vi "Melissa.vi"(9 "REPL":string, 10 "Send":string) -> ()   [LabVIEW 2020]
panel:
  in  "Serial Name":string
  out "Cover":bool
  in  "Script":string
  in  "Buffer":string
  in  "Disconnect":bool
  in  "Help":bool
  in  "Connect":bool
  in  "Stop Button":bool
  out "Running Script":bool
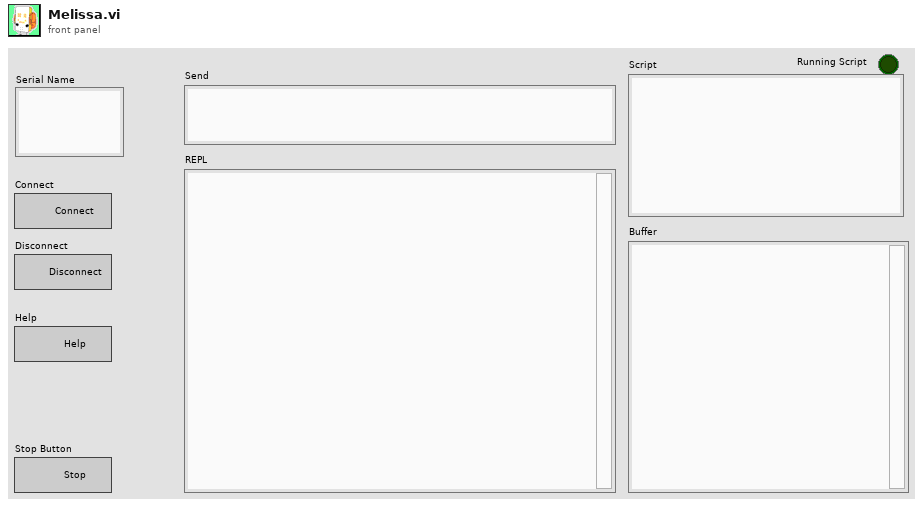
[diagram p1: front panel]
types:
  T1 = enum32{"Invalid", "Standard", "Closed", "Hidden", "Minimized", "Maximized"}
  T2 = typedef "eventvkey.ctl" = enum16{"ASCII", "Enter", "Return", "Shift", "Ctrl", "Alt", "Cmd", "Opt", "Caps", "NumLock", "Clear", "Break", "Up", "Down", "Left", "Right", "Insert", "Delete", "Home", "End", "PageUp", "PageDown", "Escape", "Help", "Pause", "ScrollLock", "F1", "F2", "F3", "F4", "F5", "F6", "F7", "F8", "F9", "F10", "F11", "F12", "F13", "F14", "F15", "F16", "F17", "F18", "F19", "F20", "F21", "F22", "F23", "F24", "Play", "VolumeUp", "VolumeDown", "Mute", "Two Byte Char"}
  T3 = cluster{"Shift":bool, "Ctrl":bool, "Alt":bool, "Cmd":bool, "Opt":bool}
  T4 = cluster{"Char":i16, "VKey":T2, "PlatMods":cluster{"Shift":bool, "Ctrl":bool, "Alt":bool, "Cmd":bool, "Opt":bool}}
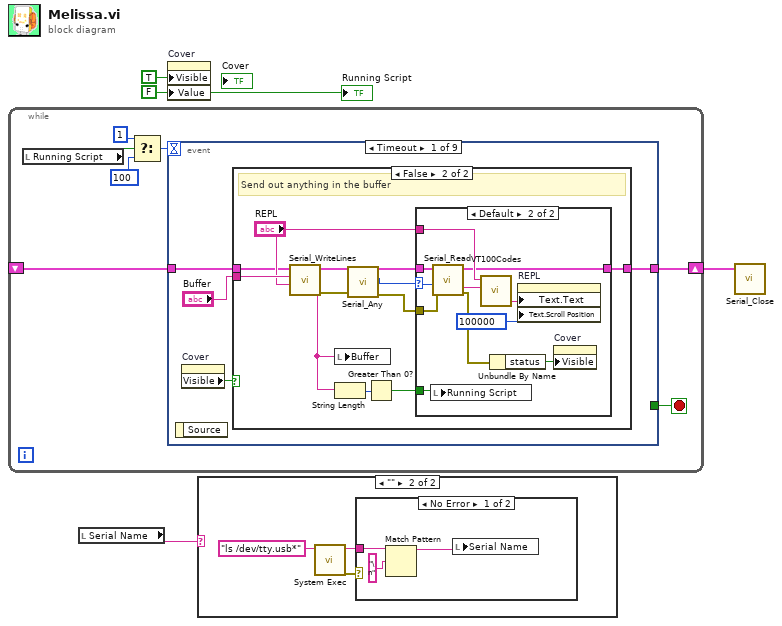
[diagram p0: block diagram]
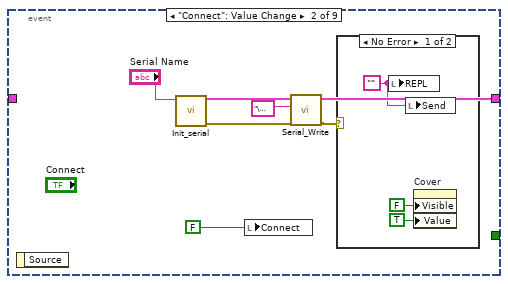
[diagram p6: hidden frame]
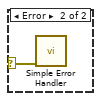
[diagram p7: hidden frame]
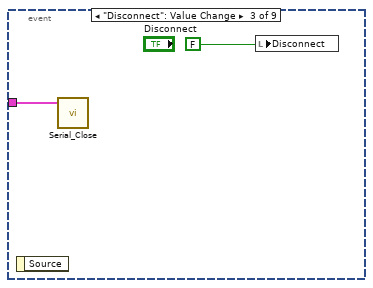
[diagram p8: hidden frame]
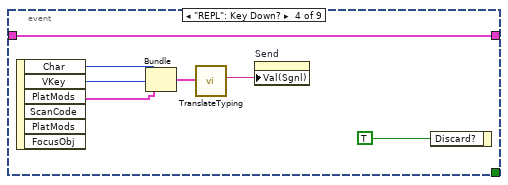
[diagram p9: hidden frame]
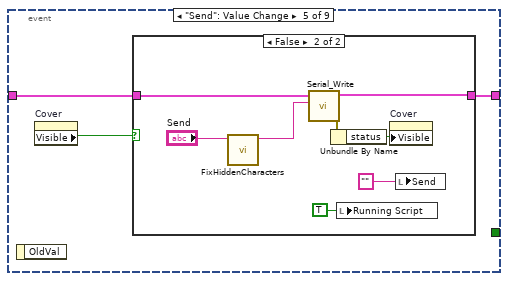
[diagram p10: hidden frame]
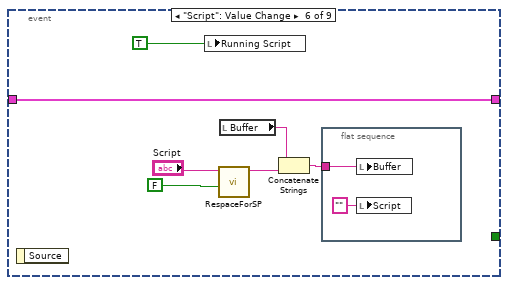
[diagram p12: hidden frame]
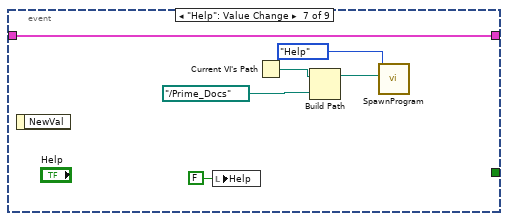
[diagram p13: hidden frame]
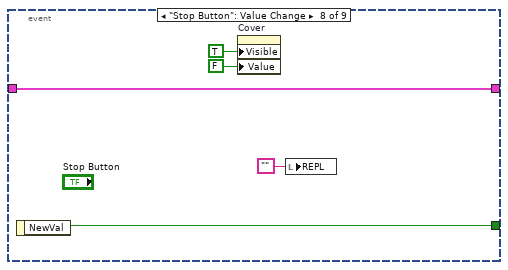
[diagram p14: hidden frame]
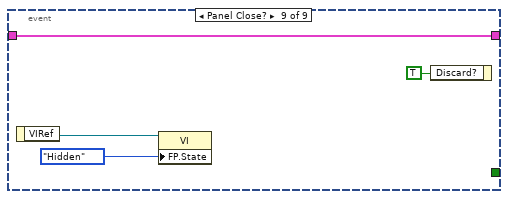
[diagram p15: hidden frame]
diagram:
  w3 = FALSE ("Cover")
  n1 = while {
    shift-right: [w10] -> w2
    shift-left: _ -> [w9]
    stop <- w11 stop-if-true
    n2 = local read "Running Script"() -> (w5:bool)
    n3 = Select(t=1, s=w5, f=100) -> (s? t:f=w6:i32)
    n4 = event shown="[0] Timeout" {
      selector: _ -> [_ _ _ _ _ _ _ _ _]
      dyn-events: _ -> [_ _ _ _ _ _ _ _ _]
      timeout: w6 -> [_ _ _ _ _ _ _ _ _]
      tunnel: [_ _ _ _ _ _ _ w90 _] -> w11
      tunnel: [w15 w41 _ w60 w62 w77 w87 w91 w96] -> w10
      tunnel: w9 -> [w14 _ w52 w60 w63 w77 w87 w91 w96]
      event Timeout {
        n5 = event-data() -> ()  [unwired: 1 in, 1 out]
        n6 = property on="Cover" class="Bool (strict)"() -> ("Visible"=w13:bool)  [unwired: 2 in, 2 out]
        n7 = case shown="False" w13 {
          tunnel: [w16 w18] -> w15
          tunnel: w14 -> [w16 w17]
          tunnel: "Buffer" -> [_ w28]
          frame True {
          }
          frame False {
            # "Send out anything in the buffer"
            n8 = call "Serial_WriteLines.vi"("REPL"="REPL", "Send"=w28, "Python in"=w17) -> ("error out"=w21:errorcluster, "Rest"=w26:string, "Python out"=w23:cluster{"Python":refnum<k35>, "py file":path})  [unwired: 6 in]
            n9 = local write "Buffer"(w26) -> ()
            n10 = String Length(string=w26) -> (length=w27:i32)
            n11 = call "Serial_Any.vi"("error in (no error)"=w21, "Python in"=w23) -> ("error out"=w20:errorcluster, "Size"=w19:i32, "Python out"=w22:cluster{"Python":refnum<k35>, "py file":path})  [unwired: 6 in, 1 out]
            n12 = Greater Than 0?(x=w27) -> (x > 0?=w25:bool)
            n13 = case shown="Default" w19 {
              selector: w19 -> [_ w30]
              tunnel: [w29 w34] -> w18
              tunnel: w22 -> [w29 w35]
              tunnel: w20 -> [_ w33]
              tunnel: w25 -> [_ w37]
              tunnel: "REPL" -> [_ w36]
              frame 0 {
              }
              frame Default {
                n14 = local write "Running Script"(w37) -> ()
                n15 = call "Serial_Read.vi"("error in (no error)"=w33, "Bytes"=w30, "Python in"=w35) -> ("error out"=w32:errorcluster, "text read"=w31:string, "Python out"=w34:cluster{"Python":refnum<k35>, "py file":path})  [unwired: 6 in]
                n16 = call "VT100Codes.vi"("read buffer"=w31, "Console In"=w36) -> ("Console Out"=w39:string)  [unwired: 9 in]
                n17 = Unbundle By Name(w32) -> ("status"=w38:bool)
                n18 = property on="REPL" class="Str"("Text.Text"=w39, "Text.Scroll Position"=u32 100000 ("Text.Selection:Start")) -> ()  [unwired: 2 in, 2 out]
                n19 = property on="Cover" class="Bool (strict)"("Visible"=w38) -> ()  [unwired: 2 in, 2 out]
              }
            }
          }
        }
      }
      event "Connect": Value Change {
        n20 = event-data() -> ()  [unwired: 1 in, 1 out]
        n21 = call "Init_serial.vi"("Serial Name"="Serial Name") -> ("error out"=w43:errorcluster, "Python out"=w44:cluster{"Python":refnum<k35>, "py file":path})  [unwired: 9 in]
        n22 = local write "Connect"(FALSE ("Help")) -> ()
        n23 = call "Serial_Write.vi"("error in (no error)"=w43, "Text to write"="\u0003" ("write buffer"), "Python in"=w44) -> ("error out"=w42:errorcluster, "Python out"=w41:cluster{"Python":refnum<k35>, "py file":path})  [unwired: 7 in]
        n24 = case shown="No Error" w42 {
          selector: w42 -> [_ w51]
          frame No Error {
            w50 = ""
            n25 = local write "REPL"(w50) -> ()
            n26 = local write "Send"(w50) -> ()
            n27 = property on="Cover" class="Bool (strict)"("Visible"=FALSE, "Value"=TRUE ("Cover")) -> ()  [unwired: 2 in, 2 out]
          }
          frame Error {
            n28 = call <vilib>:"Simple Error Handler.vi"("error in (no error)"=w51) -> ()  [unwired: 4 in, 5 out]
          }
        }
      }
      event "Disconnect": Value Change {
        n29 = event-data() -> ()  [unwired: 1 in, 1 out]
        n30 = call "Serial_Close.vi"("Python in"=w52) -> ()  [unwired: 11 in]
        n31 = local write "Disconnect"(FALSE ("Help")) -> ()
      }
      event "REPL": Key Down? {
        n32 = event-data() -> ("Char"=w56:i16, "VKey"=w57:T2, "PlatMods"=w58:T3)  [unwired: 1 in, 3 out]
        n33 = Bundle("Char"=w56, "VKey"=w57, "PlatMods"=w58) -> (w59:T4)  [unwired: 1 in]
        n34 = call "TranslateTyping.vi"("Cluster"=w59) -> ("key"=w55:string)  [unwired: 10 in]
        n35 = property on="Send" class="Str"("Val(Sgnl)"=w55) -> ()  [unwired: 2 in, 2 out]
        n36 = event-data("Discard?"=TRUE) -> ()  [unwired: 1 in, 1 out]
      }
      event "Send": Value Change {
        n37 = event-data() -> ()  [unwired: 1 in, 1 out]
        n38 = property on="Cover" class="Bool (strict)"() -> ("Visible"=w61:bool)  [unwired: 2 in, 2 out]
        n39 = case shown="False" w61 {
          tunnel: w63 -> [w64 w66]
          tunnel: [w64 w65] -> w62
          frame True {
          }
          frame False {
            n40 = call "FixHiddenCharacters.vi"("String in"="Send") -> ("String out"=w68:string)  [unwired: 10 in]
            n41 = call "Serial_Write.vi"("Text to write"=w68, "Python in"=w66) -> ("error out"=w67:errorcluster, "Python out"=w65:cluster{"Python":refnum<k35>, "py file":path})  [unwired: 8 in]
            n42 = Unbundle By Name(w67) -> ("status"=w69:bool)
            n43 = local write "Running Script"(TRUE ("Running Script")) -> ()
            n44 = property on="Cover" class="Bool (strict)"("Visible"=w69) -> ()  [unwired: 2 in, 2 out]
            n45 = local write "Send"("" ("Write text")) -> ()
          }
        }
      }
      event "Script": Value Change {
        n46 = event-data() -> ()  [unwired: 1 in, 1 out]
        n47 = local write "Running Script"(TRUE ("Visible")) -> ()
        n48 = call "RespaceForSP.vi"("Keep spaces?"=FALSE, "Code"="Script") -> ("Cleaned for SPIKE"=w74:string)  [unwired: 9 in]
        n49 = local read "Buffer"() -> (w75:string)
        n50 = Concatenate Strings(w75, w74) -> (w73:string)
        n51 = flat-sequence {
          tunnel: w73 -> [w81]
          frame #0 {
            n52 = local write "Buffer"(w81) -> ()
            n53 = local write "Script"("" ("Script")) -> ()
          }
        }
      }
      event "Help": Value Change {
        n54 = event-data() -> ()  [unwired: 1 in, 1 out]
        n55 = local write "Help"(FALSE ("Help")) -> ()
        n56 = Current VI's Path() -> (path=w85:path)
        n57 = Build Path(base path=w85, name or relative path=path "../Prime_Docs") -> (appended path=w83:path)
        n58 = call "SpawnProgram.vi"("Server"=w83, "Dialog"=enum16{"Help", "Files"}."Help") -> ()  [unwired: 10 in]
      }
      event "Stop Button": Value Change {
        n59 = event-data() -> ("NewVal"=w90:bool)  [unwired: 1 in]
        n60 = property on="Cover" class="Bool (strict)"("Visible"=TRUE, "Value"=FALSE ("Cover")) -> ()  [unwired: 2 in, 2 out]
        n61 = local write "REPL"("") -> ()
      }
      event Panel Close? {
        n62 = event-data() -> ("VIRef"=w94:refnum<vi>)  [unwired: 1 in]
        n63 = property class="VI"(reference=w94, "FP.State"=T1."Hidden" ("Front Panel Window:State")) -> ()  [unwired: 1 in, 2 out]
        n64 = event-data("Discard?"=TRUE) -> ()  [unwired: 1 in, 1 out]
      }
    }
  }
  n65 = local read "Serial Name"() -> (w1:string)
  n66 = property on="Cover" class="Bool (strict)"("Visible"=TRUE, "Value"=w3) -> ()  [unwired: 2 in, 2 out]
  n67 = case shown="\"\"" w1 {
    frame Default {
    }
    frame "" {
      n68 = call <vilib>:"System Exec.vi"("command line"="ls /dev/tty.usb*") -> ("error out"=w98:errorcluster, "standard output"=w97:string)  [unwired: 7 in, 2 out]
      n69 = case shown="No Error" w98 {
        tunnel: w97 -> [w102 _]
        frame No Error {
          n70 = Match Pattern(string=w102, regular expression="\n") -> (before substring=w100:string)  [unwired: 1 in, 3 out]
          n71 = local write "Serial Name"(w100) -> ()
        }
        frame Error {
        }
      }
    }
  }
  n72 = call "Serial_Close.vi"("Python in"=w2) -> ()  [unwired: 11 in]
  "Running Script" <- w3
